vi "IPS Set Switch Heater.vi"(4 "Error In":errorcluster={"status"=FALSE, "code"=1073676294, "source"="VISA Read in Prologix USB GPIB Command.vi"}, 6 "Switch Heater":T1, 7 "VISA resource name":refnum<visa-resource-name>="GPIB0::24::INSTR") -> (0 "Error Out":errorcluster={"status"=FALSE, "code"=1073676293, "source"="VISA Read in NI USB GPIB Command.vi->IPS Ctrl Persistent Heater.vi"}, 1 "Response":string="H\r", 3 "VISA resource name":refnum<visa-resource-name>="GPIB1::25::INSTR")   [LabVIEW 2016, in "IPS-120.lvlib"]
uses:
  IPS-120.lvlib
  Typedefs/Set Switch Heater - Enum.ctl
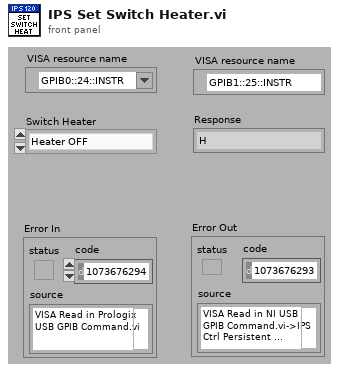
[diagram p1: front panel]
types:
  T1 = typedef "IPS-120.lvlib/Set Switch Heater - Enum.ctl" = enum16{"Heater OFF", "Heater ON if PSU=Magnet", "Heater ON, No Checks"}
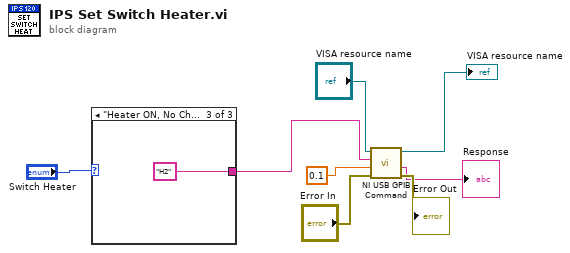
[diagram p0: block diagram]
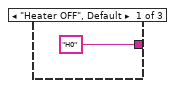
[diagram p2: hidden frame]
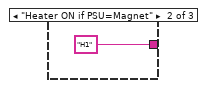
[diagram p3: hidden frame]
diagram:
  n1 = case shown="\"Heater ON, No Checks\"" "Switch Heater" {
    tunnel: ["H0" "H1" "H2"] -> w4
    frame "Heater OFF", Default {
    }
    frame "Heater ON if PSU=Magnet" {
    }
    frame "Heater ON, No Checks" {
    }
  }
  n2 = call "NI USB GPIB Command.vi"("Error In"="Error In", "Wait for instrument to respond (s)"=0.1, "String to Send"=w4, "VISA resource name"="VISA resource name") -> ("Error Out"=→"Error Out":errorcluster, "Return String from Device (Not all commands return a String)"=→"Response":string, "VISA resource name out"=→"VISA resource name":refnum<visa-resource-name>)  [unwired: 1 out]
